vi "Unescape String.vi"(11 "Escaped String":string) -> (3 "String":string)   [LabVIEW 2020, in "JSON.lvlib"]
uses:
  JSON.lvlib
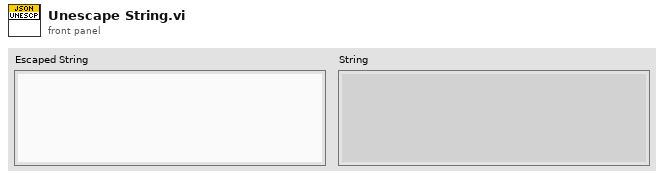
[diagram p1: front panel]
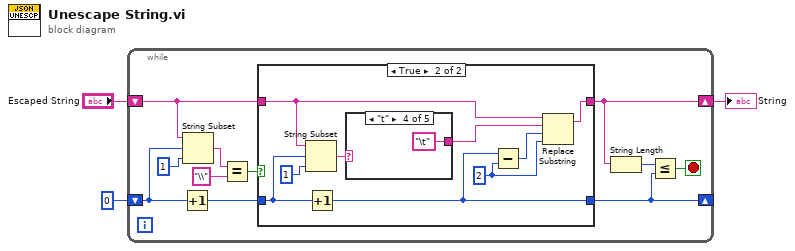
[diagram p0: block diagram]
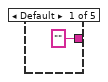
[diagram p3: hidden frame]
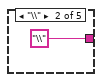
[diagram p4: hidden frame]
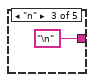
[diagram p5: hidden frame]
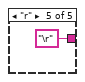
[diagram p6: hidden frame]
diagram:
  n1 = while {
    shift-right: [w7] -> w1
    shift-left: "Escaped String" -> [w9]
    shift-right: [w5] -> _
    shift-left: 0 -> [w13]
    stop <- w4 stop-if-true
    n2 = Increment(x=w13) -> (x+1=w8:i32)
    n3 = String Subset(string=w9, offset (0)=w13, length (rest)=1 ("length (rest)")) -> (substring=w12:string)
    n4 = Equal?(x=w12, y="\\") -> (x = y?=w10:bool)
    n5 = case shown="True" w10 {
      tunnel: w9 -> [w16 w18]
      tunnel: w8 -> [w15 w23]
      tunnel: [w15 w20] -> w5
      tunnel: [w16 w17] -> w7
      frame False {
      }
      frame True {
        w21 = 2 ("y")
        n6 = String Subset(string=w18, offset (0)=w23, length (rest)=1 ("length (rest)")) -> (substring=w24:string)
        n7 = Increment(x=w23) -> (x+1=w20:i32)
        n8 = case shown="\"t\"" w24 {
          tunnel: ["" ("substring (\"\")") "\\" ("substring (\"\")") "\n" ("substring (\"\")") "\t" ("substring (\"\")") "\r" ("substring (\"\")")] -> w19
          frame Default {
          }
          frame "\\" {
          }
          frame "n" {
          }
          frame "t" {
          }
          frame "r" {
          }
        }
        n9 = Subtract(x=w20, y=w21) -> (x-y=w22:i32)
        n10 = Replace Substring(2:w21, 3:w22, 4:w19, 5:w18) -> (1:w17:string)  [unwired: 1 out]
      }
    }
    n11 = String Length(string=w7) -> (length=w6:i32)
    n12 = Less Or Equal?(x=w6, y=w5) -> (x <= y?=w4:bool)
  }
  "String" <- w1
